vi "set wave.vi"(7 "file path":path, 8 "phase":i32, 9 "f":dbl=0.0078125 format="%.4e", 10 "amplitude (volts) in":dbl format="%.2f", 11 "samples":i32=128) -> (2 "amplitude (volts)":dbl format="%.2f", 3 "waveform":sgl[](array[numeric]) format="%.2f", 5 "new file path":path)   [LabVIEW 2010]
uses:
  <vilib>/Utility/file.llb/Read From Spreadsheet File (DBL).vi
  <vilib>/Analysis/NI_AALBase.lvlib
panel:
  # "ticks"
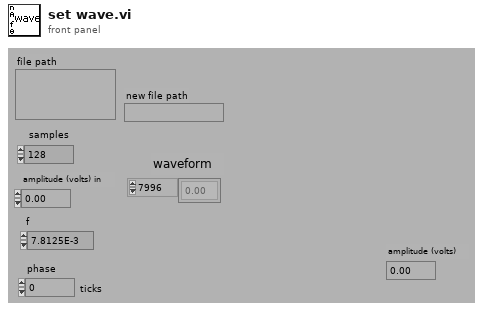
[diagram p1: front panel]
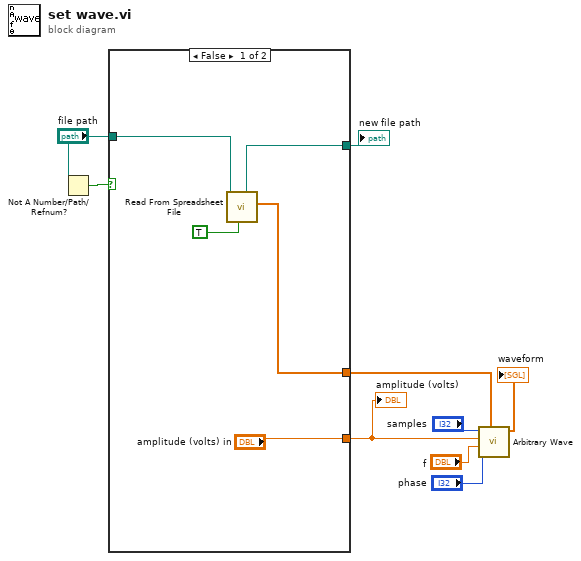
[diagram p0: block diagram]
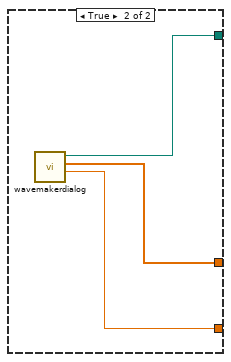
[diagram p2: hidden frame]
diagram:
  n1 = Not A Number/Path/Refnum?(number/path/refnum="file path") -> (NaN/Path/Refnum?=w2:bool)
  n2 = case shown="False" w2 {
    tunnel: [w12 w15] -> w7
    tunnel: "file path" -> [w13 _]
    tunnel: [w11 w17] -> w8
    tunnel: ["amplitude (volts) in" w16] -> w1
    frame False {
      n3 = call-poly <vilib>:"Read From Spreadsheet File.vi"("transpose (no:F)"=TRUE, "file path (dialog if empty)"=w13) -> ("first row"=w12:dbl[], "new file path (Not A Path if cancelled)"=w11:path)  [unwired: 5 in, 3 out]
    }
    frame True {
      n4 = call "wavemakerdialog.vi"() -> ("amplitude (volts)"=w16:dbl, "waveform"=w15:sgl[], "new file path"=w17:path)  [unwired: 9 in]
    }
  }
  "new file path" <- w8
  "amplitude (volts)" <- w1
  n5 = call <vilib>:"Arbitrary Wave.vi"("Wave Table"=w7, "phase in"="phase", "frequency"="f", "amplitude"=w1, "samples"="samples") -> ("arbitrary wave"=→"waveform":dbl[])  [unwired: 2 in, 2 out]
